vi "PCAN_DecompLaserPosition.vi"(0 "DATA":u8[](array[numeric])) -> (1 "Laser 1 pos.":u16, 2 "Laser 2 pos.":u16, 3 "Laser 3 pos.":u16, 4 "Laser 4 pos.":u16)   [LabVIEW 2013]
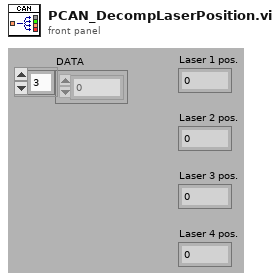
[diagram p1: front panel]
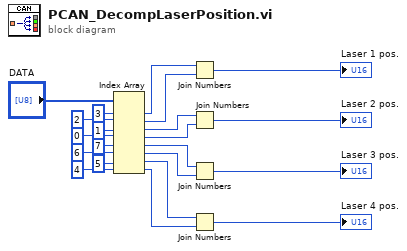
[diagram p0: block diagram]
diagram:
  n1 = Index Array(array="DATA", index #1=3 ("index"), index #2=2 ("index"), index #3=1 ("index"), index #4=0 ("index"), index #5=7 ("index"), index #6=6 ("index"), index #7=5 ("index"), index #8=4 ("index")) -> (element #1=w11:u8, element #2=w12:u8, element #3=w1:u8, element #4=w5:u8, element #5=w4:u8, element #6=w2:u8, element #7=w3:u8, element #8=w6:u8)
  n2 = Join Numbers(hi=w11, lo=w12) -> ((hi.lo)=→"Laser 1 pos.":u16)
  n3 = Join Numbers(hi=w1, lo=w5) -> ((hi.lo)=→"Laser 2 pos.":u16)
  n4 = Join Numbers(hi=w4, lo=w2) -> ((hi.lo)=→"Laser 3 pos.":u16)
  n5 = Join Numbers(hi=w3, lo=w6) -> ((hi.lo)=→"Laser 4 pos.":u16)
